vi "kPIDsatWithReset.vi"(6 "Reset":bool, 8 "PID Gains":cluster{"Kp":dbl, "Kd":dbl, "Ki":dbl}, 9 "Sat Limit":dbl, 10 "Position":dbl, 11 "Reference":dbl) -> (3 "Control":dbl)   [LabVIEW 2010, in "KevLib01.lvlib"]
uses:
  KevLib01.lvlib
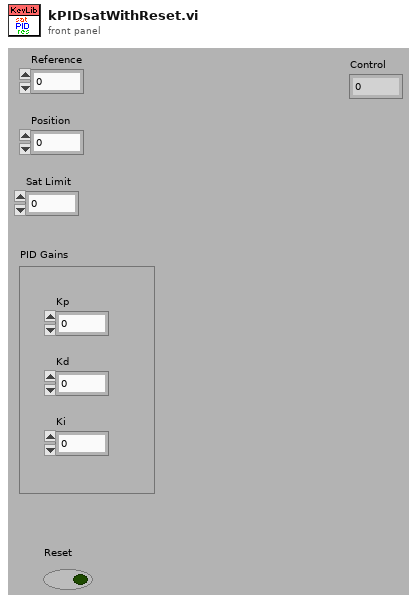
[diagram p1: front panel]
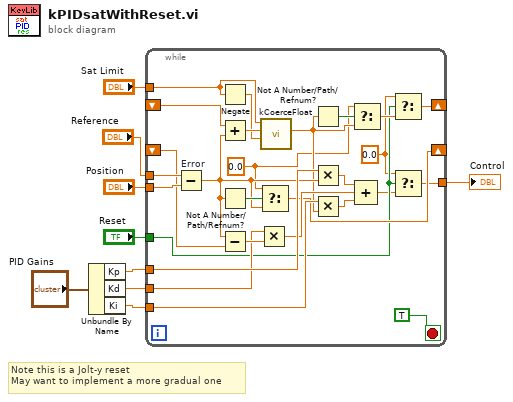
[diagram p0: block diagram]
diagram:
  # "Note this is a Jolt-y reset\nMay want to implement a more gradual one"
  n1 = Unbundle By Name("PID Gains") -> ("Kp"=w8:dbl, "Kd"=w5:dbl, "Ki"=w4:dbl)
  n2 = while {
    tunnel: w8 -> [w35]
    tunnel: "Reference" -> [w34]
    tunnel: "Position" -> [w33]
    shift-right: [w20] -> _
    shift-left: _ -> [w32]
    tunnel: w5 -> [w30]
    shift-right: [w14] -> _
    shift-left: _ -> [w29]
    tunnel: w4 -> [w28]
    tunnel: [w10] -> w3
    tunnel: "Sat Limit" -> [w23]
    tunnel: "Reset" -> [w13]
    stop <- TRUE stop-if-true
    w12 = 0.0 ("t")
    w16 = 0.0 ("t")
    n3 = Subtract "Error"(x=w34, y=w33) -> (x-y=w19:dbl)
    n4 = Negate(x=w23) -> (-x=w22:dbl)
    n5 = Add(x=w29, y=w19) -> (x+y=w24:dbl)
    n6 = Not A Number/Path/Refnum?(number/path/refnum=w19) -> (NaN/Path/Refnum?=w21:bool)
    n7 = Subtract(x=w19, y=w32) -> (x-y=w31:dbl)
    n8 = Multiply(x=w30, y=w31) -> (x*y=w26:dbl)
    n9 = Select(t=w16, s=w21, f=w19) -> (s? t:f=w20:dbl)
    n10 = call "kCoerceFloat.vi"("lower"=w22, "input"=w24, "upper"=w23) -> ("output"=w17:dbl)  [unwired: 8 out]
    n11 = Not A Number/Path/Refnum?(number/path/refnum=w17) -> (NaN/Path/Refnum?=w18:bool)
    n12 = Multiply(x=w35, y=w19) -> (x*y=w27:dbl)
    n13 = Multiply(x=w28, y=w17) -> (x*y=w25:dbl)
    n14 = Select(t=w16, s=w18, f=w17) -> (s? t:f=w15:dbl)
    n15 = Compound Arithmetic op=ADD(w27, w26, w25) -> (w11:dbl)
    n16 = Select(t=w12, s=w13, f=w15) -> (s? t:f=w14:dbl)
    n17 = Select(t=w12, s=w13, f=w11) -> (s? t:f=w10:dbl)
  }
  "Control" <- w3
